vi "BSA_Type_String.vi"(2 "BSA String in":string, 3 "BSA Type":T1) -> (0 "BSA Type Out":T1, 1 "BSA String Out":string)   [LabVIEW 2011]
uses:
  BSA_Type.ctl
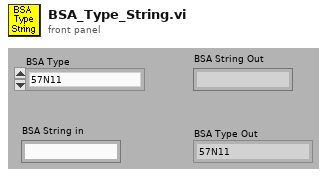
[diagram p1: front panel]
types:
  T1 = typedef "BSA_Type.ctl" = enum16{"57N11", "BSA F60"}
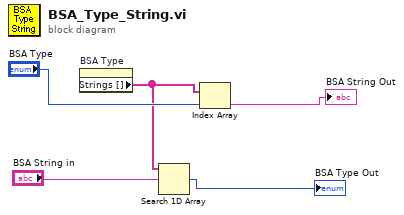
[diagram p0: block diagram]
diagram:
  n1 = property on="BSA Type" class="Enum (strict)"() -> ("Strings []"=w3:string[])  [unwired: 2 in, 2 out]
  n2 = Search 1D Array(1D array=w3, element="BSA String in") -> (index of element=→"BSA Type Out":i32)  [unwired: 1 out]
  n3 = Index Array(array=w3, index="BSA Type") -> (element=→"BSA String Out":string)
